vi "Close.vi"(2 "error in":errorcluster, 3 "AI Task in":refnum<k21>) -> (0 "error out":errorcluster)   [LabVIEW 2025]
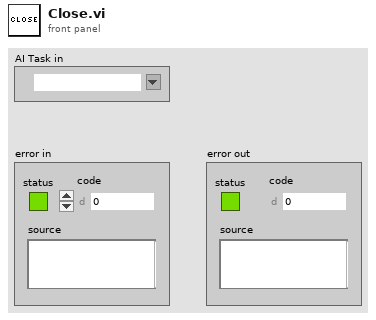
[diagram p1: front panel]
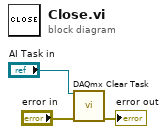
[diagram p0: block diagram]
diagram:
  n1 = call <vilib>:"DAQmx Clear Task.vi"("task in"="AI Task in", "error in"="error in") -> ("error out"=→"error out":errorcluster)  [unwired: 13 in]
